vi "Run Test.vi"(8 "error in (no error)":errorcluster, 11 "Test Template in":refnum<class "Rocom Button Test.lvclass">) -> (0 "error out":errorcluster, 1 "Fail Codes":string[](array[string]), 2 "Tests Passed":bool[](array[boolean]), 3 "Test Template out":refnum<class "Rocom Button Test.lvclass">)   [LabVIEW 2015, in "Rocom Button Test.lvclass"]
uses:
  Rocom Button Test.lvclass
  Test Class/Test Class.lvclass
  Classes/Application/Class/Application.lvclass
  Rocom Tests/Rocom Tests.lvclass
  <vilib>/Cree, Inc/Cree Test Framework/Classes/Base Objects/Base Class/Base Class/Base Class.lvclass
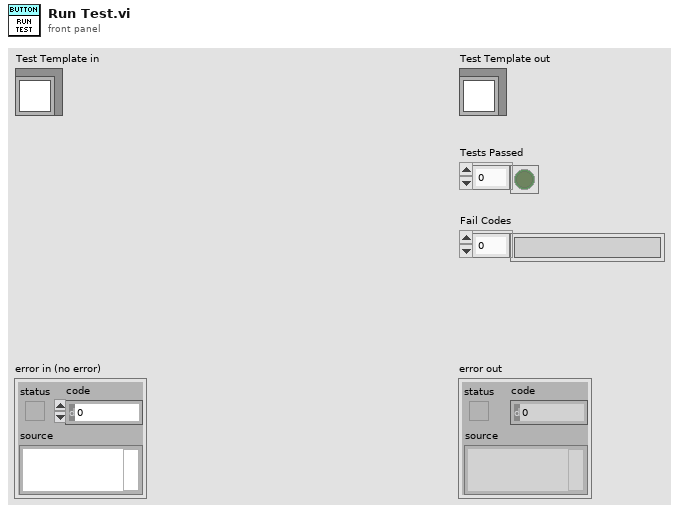
[diagram p1: front panel]
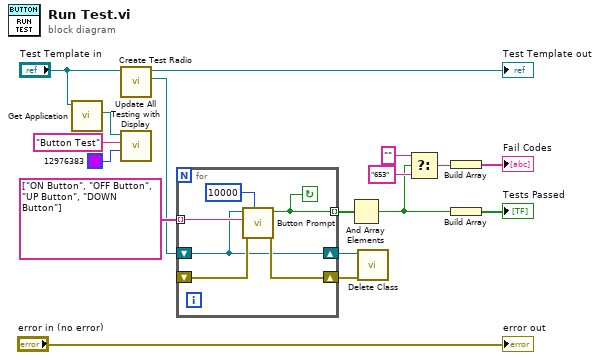
[diagram p0: block diagram]
diagram:
  n1 = call "Get Application.vi"("Test Class in"="Test Template in") -> ("Application.lvlib:Application.lvclass"=w13:refnum<class "Application.lvclass">)  [unwired: 9 in, 1 out]
  n2 = call "Create Test Radio.vi"("Rocom Tests in"="Test Template in") -> ("Test Radio"=w5:refnum<class "SC Manufacturing Test.lvclass">, "Rocom Tests out"=→"Test Template out":refnum<class "Rocom Button Test.lvclass">)  [unwired: 8 in, 1 out]
  n3 = call "Update All Testing with Display.vi"("BG Color"=u32 12976383, "Message ('')"="Button Test", "Application in"=w13) -> ()  [unwired: 7 in, 2 out]
  n4 = for {
    tunnel: string[] ["ON Button", "OFF Button", "UP Button", "DOWN Button"] ("Button to Check") -> [w21] mode=indexing
    shift-right: [w20] -> w2
    shift-left: w5 -> [w20]
    shift-right: [w22] -> w1
    shift-left: _ -> [w23]
    tunnel: [w18] -> w4 mode=indexing
    stop <- w18 continue-if-true
    n5 = call "Button Prompt.vi"("Timeout"=10000, "Error in"=w23, "Button to Check"=w21, "TestRadio"=w20) -> ("Error out"=w22:errorcluster, "Pass"=w18:bool)  [unwired: 6 in]
  }
  n6 = And Array Elements(Boolean array=w4) -> (logical AND=w3:bool)
  n7 = call <vilib>:"Delete Class.vi"("error in (no error)"=w1, "Base Class in"=w2) -> ()  [unwired: 8 in, 2 out]
  n8 = Select(t="", s=w3, f="653") -> (s? t:f=w17:string)
  n9 = Build Array(w17) -> (→"Fail Codes":string[])
  n10 = Build Array(w3) -> (→"Tests Passed":bool[])
  "error out" <- "error in (no error)"
